vi "Compteur.vi"(8 "error in (no error)":errorcluster, 11 "Machine d'état in":refnum<class "Machine d'état.lvclass">) -> (0 "error out":errorcluster, 3 "Machine d'état out":refnum<class "Machine d'état.lvclass">)   [LabVIEW 2020, in "Machine d'état.lvlib" / "Machine d'état.lvclass"]
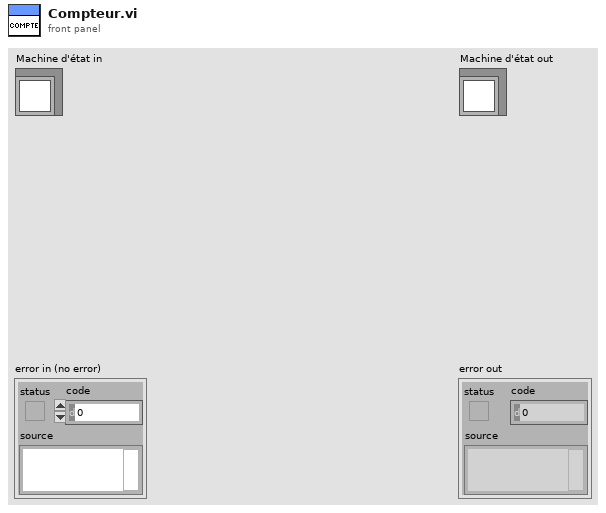
[diagram p1: front panel]
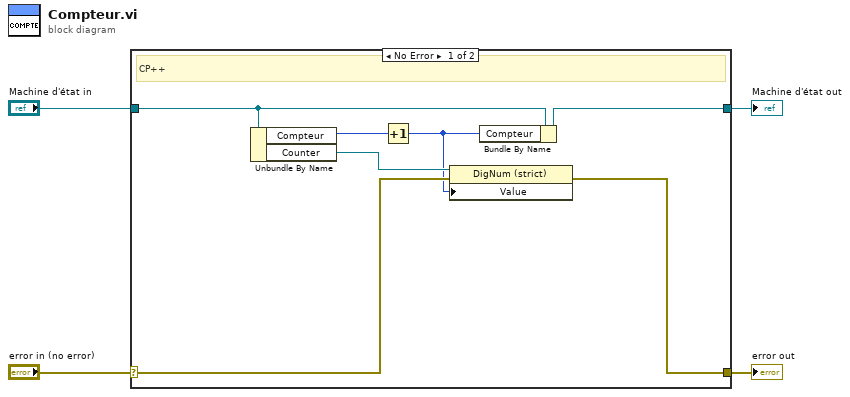
[diagram p0: block diagram]
diagram:
  n1 = case shown="No Error" "error in (no error)" {
    selector: "error in (no error)" -> [w8 w13]
    tunnel: [w7 w13] -> w3
    tunnel: [w11 w12] -> w1
    tunnel: "Machine d'état in" -> [w10 w12]
    frame No Error {
      # "CP++"
      n2 = Unbundle By Name(w10) -> ("Compteur"=w9:u8, "Counter"=w6:refnum<vi>)
      n3 = Increment(x=w9) -> (x+1=w5:u8)
      n4 = property class="DigNum (strict)"(reference=w6, error in=w8, "Value"=w5) -> (error out=w7:errorcluster)  [unwired: 1 out]
      n5 = Bundle By Name(cluster=w10, "Compteur"=w5) -> (w11:refnum<class "Machine d'état.lvclass">)
    }
    frame Error {
    }
  }
  "error out" <- w3
  "Machine d'état out" <- w1
